vi "Text_Base_Comm.vi"() -> ()   [LabVIEW 2013]
panel:
  in  "file path":path
  out "Array":errorcluster[](array[cluster])
  out "standard output":string
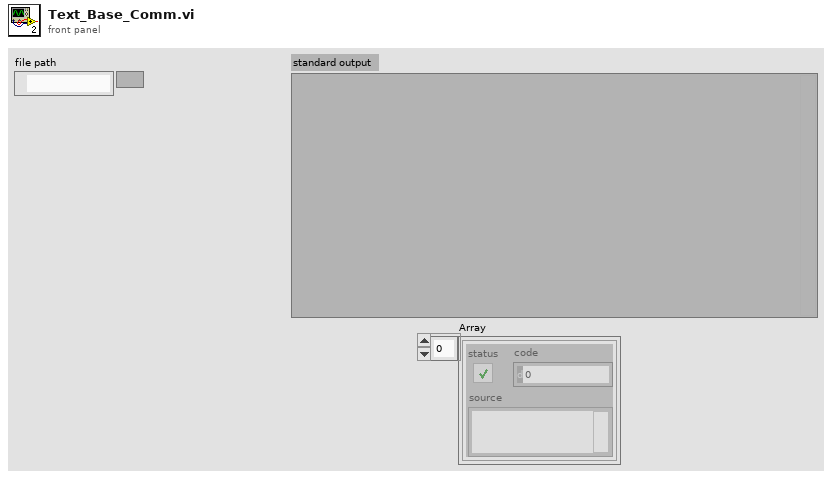
[diagram p1: front panel]
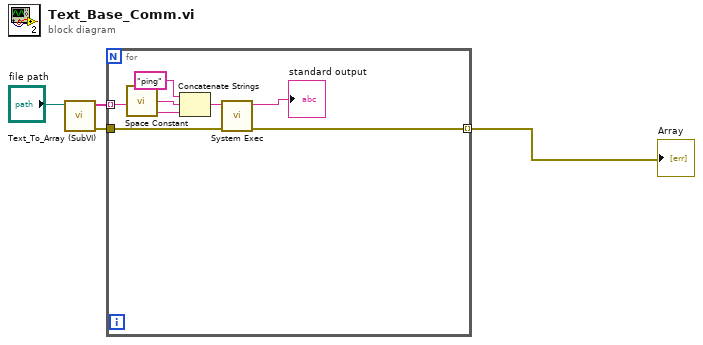
[diagram p0: block diagram]
diagram:
  n1 = call "Text_To_Array (SubVI).vi"("file path"="file path") -> ("error out"=w3:errorcluster, "Array"=w4:string[])  [unwired: 9 in]
  n2 = for {
    tunnel: w4 -> [w7] mode=indexing
    tunnel: w3 -> [w10]
    tunnel: [w9] -> w2 mode=indexing
    n3 = call <vilib>:"Space Constant.vi"() -> ("String"=w5:string)
    n4 = Concatenate Strings("ping", w5, w7) -> (w8:string)
    n5 = call <vilib>:"System Exec.vi"("error in (no error)"=w10, "command line"=w8) -> ("error out"=w9:errorcluster, "standard output"=→"standard output":string)  [unwired: 6 in, 2 out]
  }
  "Array" <- w2
